vi "Measure FPGA pulse width.vi"(8 "error in (no error)":errorcluster) -> (0 "error out":errorcluster, 3 "Numeric":dbl)   [LabVIEW 2013]
uses:
  <vilib>/DAQmx/read.llb/DAQmx Read (Counter DBL 1Chan 1Samp).vi
  <vilib>/DAQmx/create/channels.llb/DAQmx Create Channel (CI-Pulse Width).vi
  <vilib>/DAQmx/miscellaneous.llb/DAQmx Fill In Error Info.vi
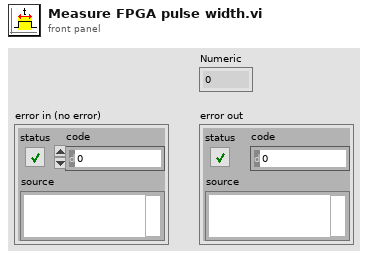
[diagram p1: front panel]
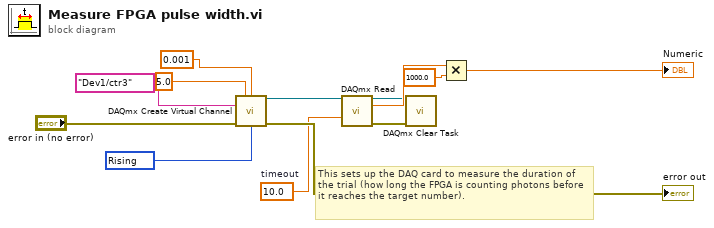
[diagram p0: block diagram]
diagram:
  w9 = 10.0  # timeout
  w5 = 10280 items=["Rising"=10280, "Falling"=10171] ("Starting Edge")
  # "This sets up the DAQ card to measure the duration of the trial (how long the FPGA is counting photons before it reaches the target number)."
  n1 = call-poly <vilib>:"DAQmx Create Virtual Channel.vi"("maximum value"=5.0 ("Maximum Value (sec)"), "minimum value"=0.001 ("Minimum Value (sec)"), "counter"=tag "Dev1/ctr3" ("Physical Channel"), "error in"="error in (no error)", "starting edge"=w5) -> ("task out"=w4:refnum<k21>, "error out"=→"error out":errorcluster)  [unwired: 9 in]
  n2 = call-poly <vilib>:"DAQmx Read.vi"("task/channels in"=w4, "timeout"=w9) -> ("task out"=w6:refnum<k21>, "data"=w11:dbl, "error out"=w7:errorcluster)  [unwired: 11 in]
  n3 = call <vilib>:"DAQmx Clear Task.vi"("task in"=w6, "error in"=w7) -> ()  [unwired: 13 in, 1 out]
  n4 = Multiply(x=w11, y=1000.0) -> (x*y=→"Numeric":dbl)
